vi "PickModel.vi"(8 "error in":errorcluster, 10 "position in":T1, 11 "class data in":refnum<class "SceneRoot.lvclass">) -> (0 "error out":errorcluster, 2 "picked out":cluster{"Node Path":refnum<vi>[]}[](array[cluster]), 3 "class data out":refnum<class "SceneRoot.lvclass">)   [LabVIEW 2010, in "RenderBase.lvlib" / "SceneRoot.lvclass"]
doc: "Picks objects at the given position from the scene."
uses:
  SceneRoot.lvclass
  <vilib>/Utility/miscctls.llb/LVPoint32TypeDef.ctl
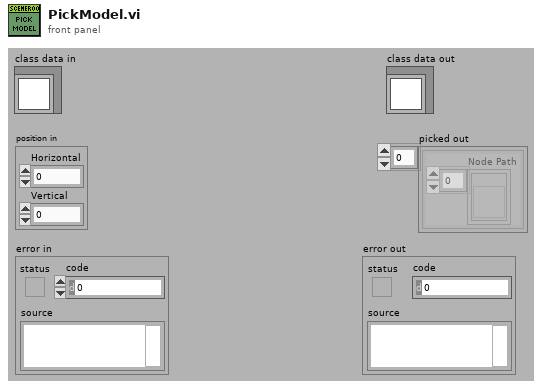
[diagram p1: front panel]
types:
  T1 = typedef "LVPoint32TypeDef.ctl" = cluster{"Horizontal":i32, "Vertical":i32}
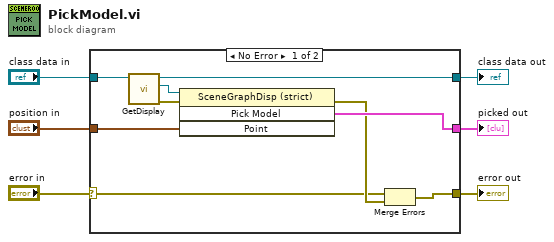
[diagram p0: block diagram]
diagram:
  n1 = case shown="No Error" "error in" {
    selector: "error in" -> [w7 w16]
    tunnel: "position in" -> [w15 _]
    tunnel: [w14 _] -> w5
    tunnel: "class data in" -> [w13 w17]
    tunnel: [w8 w16] -> w3
    tunnel: [w9 w17] -> w2
    frame No Error {
      n2 = call "GetDisplay.vi"("reference in"=w13) -> ("error out"=w11:errorcluster, "Display"=w10:refnum<vi>, "reference out"=w9:refnum<class "SceneRoot.lvclass">)  [unwired: 8 in]
      n3 = invoke on="Invoke Node" class="SceneGraphDisp (strict)" method="Pick Model"(reference=w10, error in=w11, "Point"=w15) -> (error out=w12:errorcluster, "Pick Model"=w14:cluster{"Node Path":refnum<vi>[]}[])  [unwired: 1 in, 2 out]
      n4 = Merge Errors(w7, w12) -> (w8:errorcluster)
    }
    frame Error {
    }
  }
  "picked out" <- w5
  "error out" <- w3
  "class data out" <- w2
